vi "ParseArgumentsCore.vi"(8 "error in (no error)":errorcluster, 9 "Value":string, 10 "Option":string, 11 "ExecuteBuildSpecAllTargets in":refnum<class "ExecuteBuildSpecAllTargets.lvclass">) -> (0 "error out":errorcluster, 3 "ExecuteBuildSpecAllTargets out":refnum<class "ExecuteBuildSpecAllTargets.lvclass">)   [LabVIEW 2014, in "ExecuteBuildSpecAllTargets.lvclass"]
uses:
  ExecuteBuildSpecAllTargets.lvclass
  <nishared>/LabVIEW CLI/Operations/Utilities/OperationErrorType.ctl
  ExecuteBuildSpecAllTargets.lvclass/ExecuteBuildSpecAllTargets.ctl
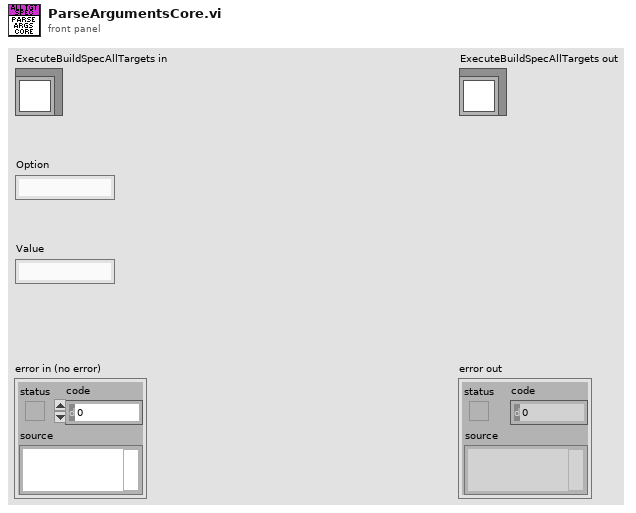
[diagram p1: front panel]
types:
  T1 = typedef "OperationErrorType.ctl" = enum16{"RequiredArgumentMissing", "UnknownArguments", "LoggerSetMultipleTimes", "OperationBrokenError"}
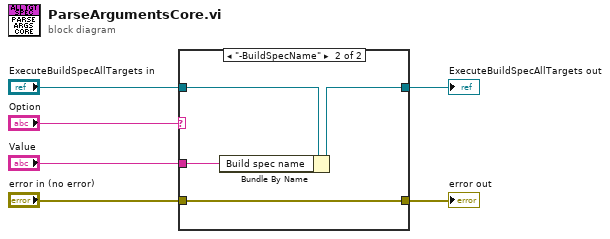
[diagram p0: block diagram]
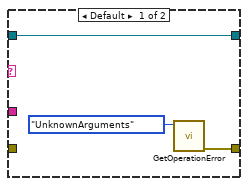
[diagram p2: hidden frame]
diagram:
  n1 = case shown="\"-BuildSpecName\"" "Option" {
    tunnel: "error in (no error)" -> [_ w13]
    tunnel: [w7 w13] -> w2
    tunnel: "Value" -> [_ w12]
    tunnel: "ExecuteBuildSpecAllTargets in" -> [w9 w11]
    tunnel: [w9 w10] -> w3
    frame Default {
      n2 = call <nishared>:"GetOperationError.vi"("Operation Error Type"=OperationErrorType."UnknownArguments") -> ("error out"=w7:errorcluster)  [unwired: 10 in]
    }
    frame "-BuildSpecName" {
      n3 = Bundle By Name(cluster=w11, "Build spec name"=w12) -> (w10:refnum<class "ExecuteBuildSpecAllTargets.lvclass">)
    }
  }
  "error out" <- w2
  "ExecuteBuildSpecAllTargets out" <- w3
